vi "Setup Menu Bar.vi"(8 "error in (no error)":errorcluster, 11 "menu reference":refnum<k9>) -> (0 "error out":errorcluster)   [LabVIEW 2017, in "Application Manager.lvclass"]
doc: "Setup the front panel's Menu Bar"
uses:
  Application Manager.lvclass
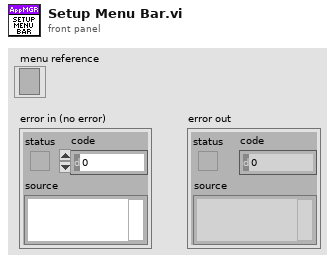
[diagram p1: front panel]
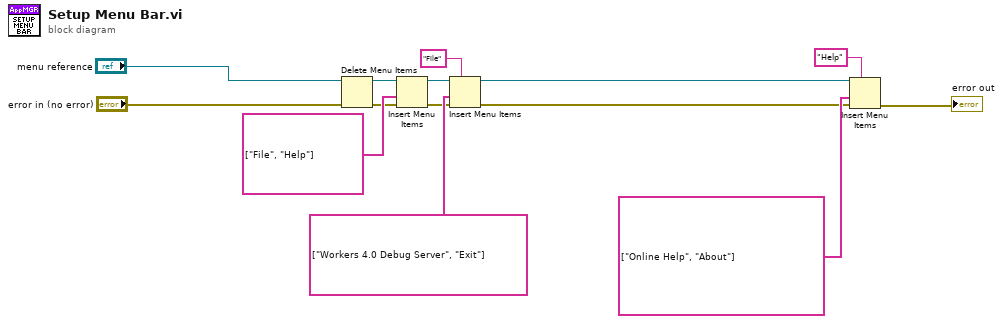
[diagram p0: block diagram]
diagram:
  n1 = Delete Menu Items(6:"error in (no error)", 9:"menu reference") -> (0:w8:errorcluster, 3:w9:refnum<k9>)  [unwired: 2 in]
  n2 = Insert Menu Items(6:w8, 7:string[] ["File", "Help"] ("L10n_item tags 1"), 9:w9) -> (0:w12:errorcluster, 3:w13:refnum<k9>)  [unwired: 3 in, 1 out]
  n3 = Insert Menu Items(5:"File" ("L10n_menu tag"), 6:w12, 7:string[] ["Workers 4.0 Debug Server", "Exit"] ("L10n_item tags 2"), 9:w13) -> (0:w2:errorcluster, 3:w3:refnum<k9>)  [unwired: 2 in, 1 out]
  n4 = Insert Menu Items(5:"Help" ("menu tag"), 6:w2, 7:string[] ["Online Help", "About"] ("L10n_item tags 2"), 9:w3) -> (0:→"error out":errorcluster)  [unwired: 2 in, 2 out]
